vi "DualDigitalOscilloscope.vi"() -> ()   [LabVIEW 2014]
panel:
  out "error out":errorcluster
  in  "Digitizing Parameters":T1
  in  "Stop Button":bool
  out "Waveform Graph":dynamicdata(graph)
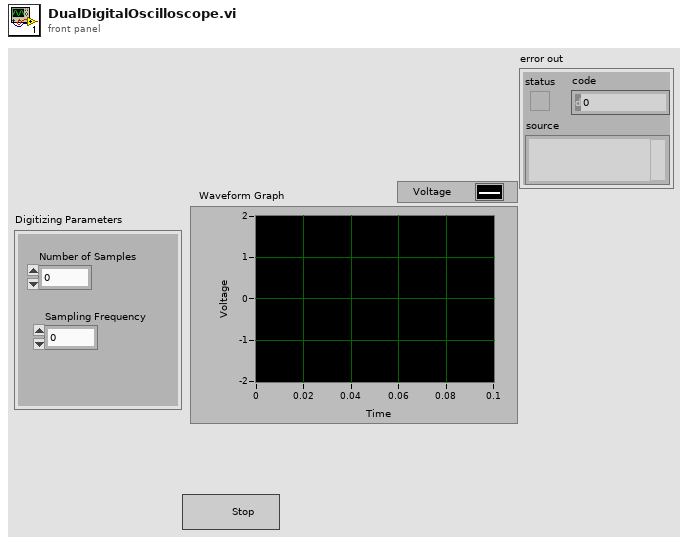
[diagram p1: front panel]
types:
  T1 = cluster{"Number of Samples":dbl, "Sampling Frequency":dbl}
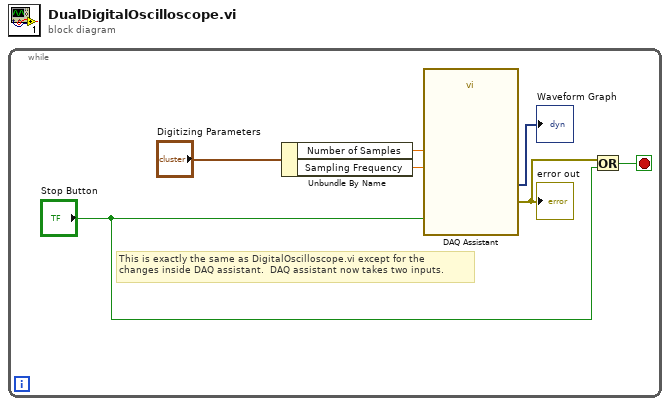
[diagram p0: block diagram]
diagram:
  n1 = while {
    stop <- w1 stop-if-true
    # "This is exactly the same as DigitalOscilloscope.vi except for the \nchanges inside DAQ assistant.  DAQ assistant now takes two inputs."
    n2 = Unbundle By Name("Digitizing Parameters") -> ("Number of Samples"=w6:dbl, "Sampling Frequency"=w5:dbl)
    n3 = call "DAQ Assistant"("rate"=w5, "number of samples"=w6, "stop (T)"="Stop Button") -> ("data"=→"Waveform Graph":dynamicdata, "error out"=w3:errorcluster)  [unwired: 14 in, 1 out]
    "error out" <- w3
    n4 = Or(x=w3, y="Stop Button") -> (x .or. y?=w1:bool)
  }
